vi "Close_Comm.vi"(8 "error in (no error)":errorcluster, 11 "Serial Port in":refnum<visa-resource-name>) -> (0 "error out":errorcluster)   [LabVIEW 2015, in "Chemyx_Syringe_Pump_driver.lvlib"]
doc: "Closes communication on the serial port."
uses:
  Chemyx_Syringe_Pump_driver.lvlib
panel:
  # "Closes communication on the serial port."
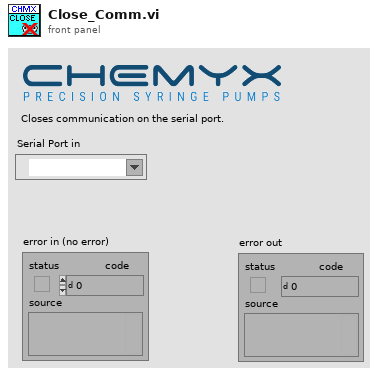
[diagram p1: front panel]
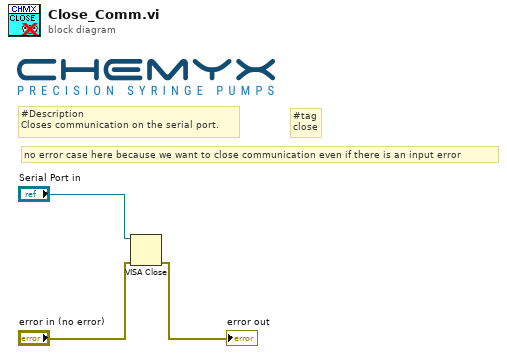
[diagram p0: block diagram]
diagram:
  # "#tag\nclose"
  # "no error case here because we want to close communication even if there is an input error"
  # "#Description\nCloses communication on the serial port."
  n1 = VISA Close(VISA resource name="Serial Port in", error in (no error)="error in (no error)") -> (error out=→"error out":errorcluster)
